vi "Obtain Session.vi"(0 "PropertyObject":refnum<k7>, 11 "error in (no error)":errorcluster) -> (4 "Session Handle":T1, 15 "error out":errorcluster)   [LabVIEW 2020, in "HTS.lvlib" / "VariableContainer.lvclass"]
doc: "This function initializes the measurement\n\nPass the function a name to obtain an active measurement handle"
uses:
  VariableContainer.lvclass
  Typedefs/Session Handle.ctl
  C:/Program Files (x86)/National Instruments/LabVIEW 2020/user.lib/_Session Fwk/Session - Root.lvclass
  VariableContainer.lvclass/VariableContainer.ctl
  <userlib>/_Session Fwk/Session - Root.lvclass
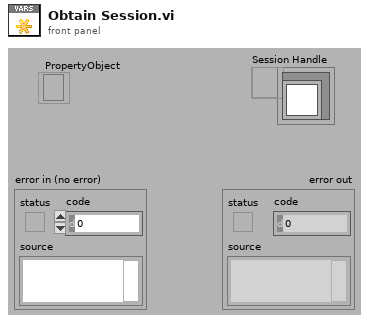
[diagram p1: front panel]
types:
  T1 = typedef "HTS.lvlib/VariableContainer.lvclass/Session Handle.ctl" = refnum<data-value>
  T2 = typedef "Session - Root.lvclass/Session Handle.ctl" = refnum<data-value>
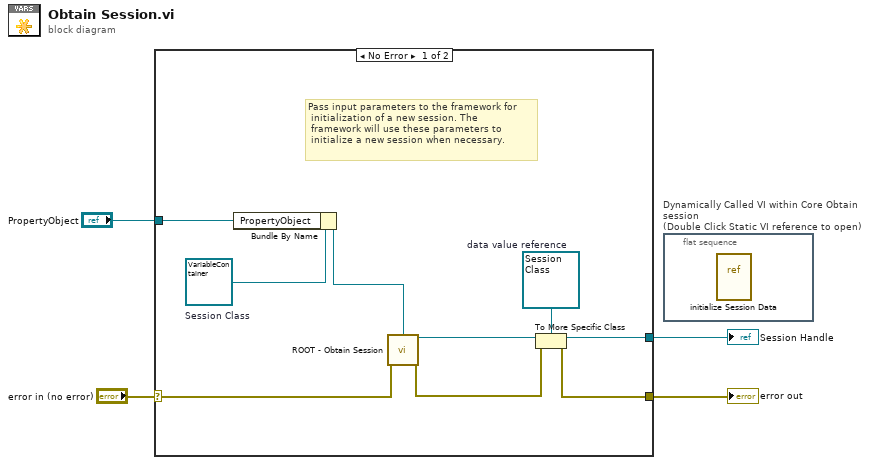
[diagram p0: block diagram]
diagram:
  n1 = case shown="No Error" "error in (no error)" {
    selector: "error in (no error)" -> [w13 w14]
    tunnel: [w10 w14] -> w3
    tunnel: [w12 _] -> w2
    tunnel: "PropertyObject" -> [w7 _]
    frame No Error {
      w5 = refnum<data-value> refnum  # data value reference
      w6 = refnum<class "VariableContainer.lvclass"> refnum  # Session Class
      # "Pass input parameters to the framework for\n initialization of a new session. The\n framework will use these parameters to\n initialize a new session when necessary."
      n2 = Bundle By Name(cluster=w6, "PropertyObject"=w7) -> (w8:refnum<class "VariableContainer.lvclass">)
      n3 = call <userlib>:"ROOT - Obtain Session.vi"("OBJ - Session"=w8, "error in (no error)"=w13) -> ("Session Handle"=w9:T2, "error out"=w11:errorcluster)  [unwired: 11 in, 1 out]
      n4 = To More Specific Class(target class=w5, reference=w9, error in=w11) -> (specific class reference=w12:refnum<data-value>, error out=w10:errorcluster)
    }
    frame Error {
    }
  }
  "error out" <- w3
  "Session Handle" <- w2
  n5 = flat-sequence "Dynamically Called VI within Core Obtain session\n(Double Click Static VI reference to open)" {
    frame #0 {
      n6 = vi-ref "initialize Session Data.vi"() -> ()  [unwired: 1 out]
    }
  }
